vi "test_4_2(SubVI).vi"(0 "Voltage":dbl, 5 "y":i32=100, 7 "Lux function":dbl, 9 "Numeric":i32, 11 "Filename":path=path "C:/Users/Dyakov_AVi/Nextcloud/bioreactor_labview/test_1.lvm") -> ()   [LabVIEW 2016]
uses:
  <vilib>/express/express shared/transition.llb/Dynamic To Waveform Array.vi
  <vilib>/express/express signal manip/GetorSetDDTAttributes/Set DDT Attributes/SetT0.vi
  <vilib>/express/express shared/transition.llb/Waveform Array To Dynamic.vi
  <vilib>/express/express signal manip/GetorSetDDTAttributes/Set DDT Attributes/Set DDT Properties.xnode
  <vilib>/ptbypt/NI_PtbyPt.lvlib
panel:
  out "hour":i32
  out "minute":i32
  out "second":i32
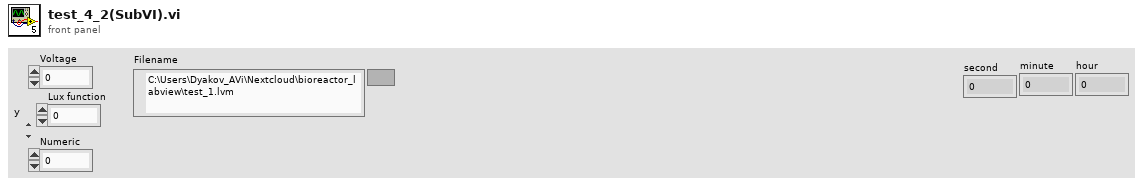
[diagram p1: front panel]
types:
  T1 = typedef "LVDateTimeRec.ctl" = cluster{"fractional second":dbl, "second":i32, "minute":i32, "hour":i32, "day of month":i32, "month":i32, "year":i32, "day of week":i32, "day of year":i32, "DST":i32}
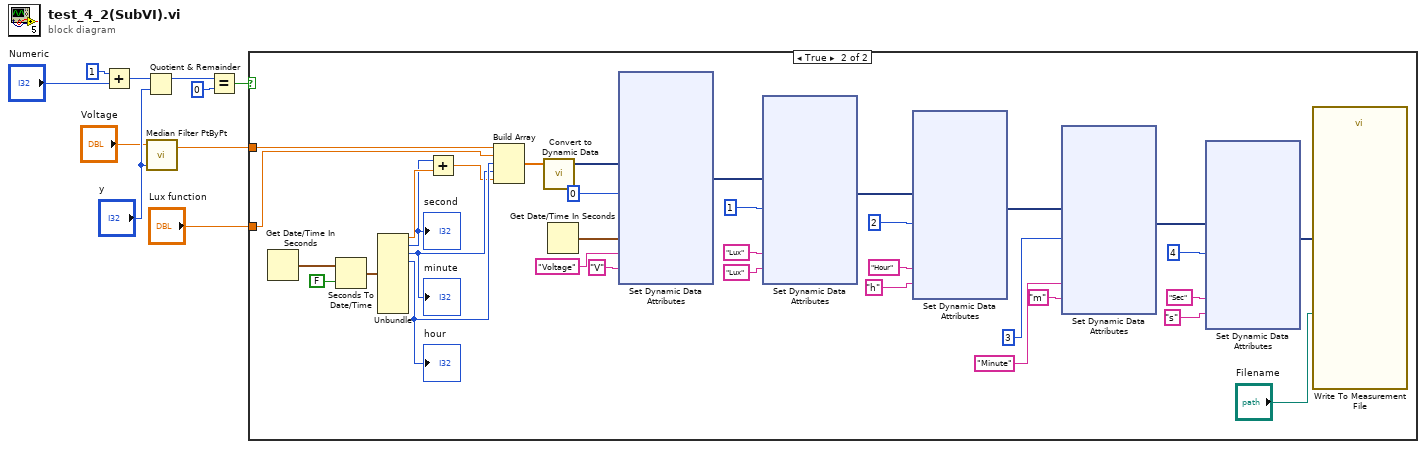
[diagram p0: block diagram]
diagram:
  n1 = Add(x=1, y="Numeric") -> (x+y=w7:i32)
  n2 = Quotient & Remainder(x=w7, y="y") -> (x-y*floor(x/y)=w4:i32)  [unwired: 1 out]
  n3 = call <vilib>:"Median Filter PtByPt.vi"("rank"="y", "x"="Voltage") -> ("Filtered x"=w1:dbl)  [unwired: 2 in, 1 out]
  n4 = Equal?(x=w4, y=0) -> (x = y?=w10:bool)
  n5 = case shown="True" w10 {
    tunnel: w1 -> [_ w43]
    tunnel: "Lux function" -> [_ w15]
    frame False {
    }
    frame True {
      n6 = Get Date/Time In Seconds() -> (seconds since 1Jan1904=w28:timestamp)
      n7 = Seconds To Date/Time(time stamp (now)=w28, to UTC (F)=FALSE) -> (date time rec=w31:T1)
      n8 = Unbundle(w31) -> ("fractional second"=w14:dbl, "second"=w13:i32, "minute"=w26:i32, "hour"=w27:i32)  [unwired: 6 out]
      "second" <- w13
      "minute" <- w26
      "hour" <- w27
      n9 = Add(x=w13, y=w14) -> (x+y=w12:dbl)
      n10 = Build Array(w43, w15, w27, w26, w12) -> (w42:dbl[])
      n11 = call "Convert to Dynamic Data"("Array"=w42) -> ("Dynamic Data Type"=w32:dynamicdata)  [unwired: 3 in]
      n12 = Get Date/Time In Seconds() -> (seconds since 1Jan1904=w30:timestamp)
      n13 = xnode "Set Dynamic Data Attributes"("Signals In"=w32, "Signal Index"=0, "Timestamp"=w30, "Signal Name"="Voltage", "Unit"="V") -> ("Signals Out"=w41:dynamicdata)  [unwired: 1 in, 1 out]
      n14 = xnode "Set Dynamic Data Attributes"("Signals In"=w41, "Signal Index"=1, "Signal Name"="Lux", "Unit"="Lux") -> ("Signals Out"=w38:dynamicdata)  [unwired: 1 in, 1 out]
      n15 = xnode "Set Dynamic Data Attributes"("Signals In"=w38, "Signal Index"=2, "Signal Name"="Hour", "Unit"="h") -> ("Signals Out"=w37:dynamicdata)  [unwired: 1 in, 1 out]
      n16 = xnode "Set Dynamic Data Attributes"("Signals In"=w37, "Signal Index"=3, "Signal Name"="Minute", "Unit"="m") -> ("Signals Out"=w36:dynamicdata)  [unwired: 1 in, 1 out]
      n17 = xnode "Set Dynamic Data Attributes"("Signals In"=w36, "Signal Index"=4, "Signal Name"="Sec", "Unit"="s") -> ("Signals Out"=w11:dynamicdata)  [unwired: 1 in, 1 out]
      n18 = call "Write To Measurement File"("Signals"=w11, "Filename"="Filename") -> ()  [unwired: 15 in, 3 out]
    }
  }
